vi "numCmd_Recv_Chassis.vi"(7 "Command Name":string, 11 "Initial Chassis Speeds":T1 {"vOmega" format="%10.3f"; "vY" format="%10.3f"; "vX" format="%10.3f"}) -> (0 "error out":errorcluster, 2 "Any Changed":bool, 3 "Chassis Speeds":T1 {"vOmega" format="%10.3f"; "vY" format="%10.3f"; "vX" format="%10.3f"})   [LabVIEW 2019, in "Trajectory_Library.lvlib"]
uses:
  Trajectory_Library.lvlib
  TypeDef/CHASSIS_SPEEDS.ctl
  numCmd_ObtainQueue_Generic.vi
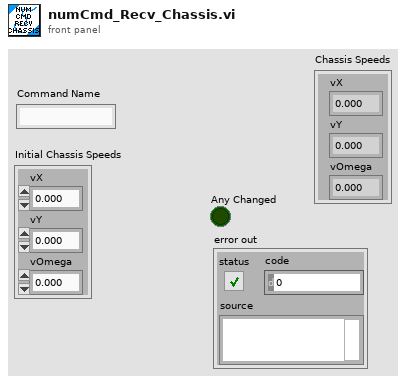
[diagram p1: front panel]
types:
  T1 = typedef "Trajectory_Library.lvlib/CHASSIS_SPEEDS.ctl" = cluster{"vX":dbl, "vY":dbl, "vOmega":dbl}
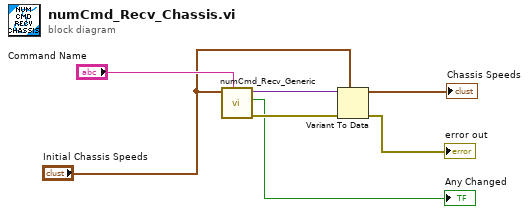
[diagram p0: block diagram]
diagram:
  n1 = call "numCmd_Recv_Generic.vi"("Command Name"="Command Name", "Initial Value"="Initial Chassis Speeds") -> ("error out"=w7:errorcluster, "Changed"=→"Any Changed":bool, "Newest Value"=w2:variant)  [unwired: 7 in]
  n2 = Variant To Data(error in=w7, type="Initial Chassis Speeds", Variant=w2) -> (data=→"Chassis Speeds":T1, error out=→"error out":errorcluster)
